vi "运维调试_总磷总氮.vi"() -> ()   [LabVIEW 2016, in "斯坦道总磷总氮.lvlib"]
uses:
  <vilib>/Utility/miscctls.llb/LVPointTypeDef.ctl
  <vilib>/Plasmionique/MB Master/MB_Master/MB_Master.lvclass
  <vilib>/ptbypt/NI_PtbyPt.lvlib
panel:
  out "步骤":u16
  out "seconds since 1Jan1904 2":timestamp
  out "seconds since 1Jan1904":timestamp
  in  "周期设置":bool
  in  "流程操作":bool
  out "消解压力":sgl format="%#.2f kPa"
  out "权限等级":string
  out "总步数":i32
  out "滑动杆":dbl(slide) caption="测试进度" scale=0.0..100.0
  out "试剂余量显示":sgl[][](graph)
  in  "仪器校准":bool
  in  "参数查询":bool
  out "简易步骤名称":string
  in  "温度曲线":bool
  in  "试剂余量":bool
  in  "灯值调整":bool
  out "固件版本号":string
  out "模块版本号":string
  out "注射器温度":sgl format="%#.2f ℃"
  out "消解温度":sgl format="%#.2f ℃"
  out "ADC":sgl
  out "F3":sgl format="%#.6f"
  out "F2":sgl format="%#.6f"
  out "F1":sgl format="%#.6f"
  out "F0":sgl format="%#.6f"
  out "运行状态":T1 {"数据时间:" format="%<%y/%m/%d %H:%M:%S>T"; "仪器时间:" format="%<%y/%m/%d %H:%M:%S>T"}
  in  "单选按钮":T2=enum."总氮"
  in  "布尔":bool
  in  "外设固件":bool
  out "字符串 2":string
  in  "数组":string[](array[string])
  in  "返回":bool
  in  "参数设置":bool
  out "集成报警信息":string
  in  "停止":bool
  in  "手动启动":bool
  in  "调试":bool
  out "多列列表框":i32(listbox)
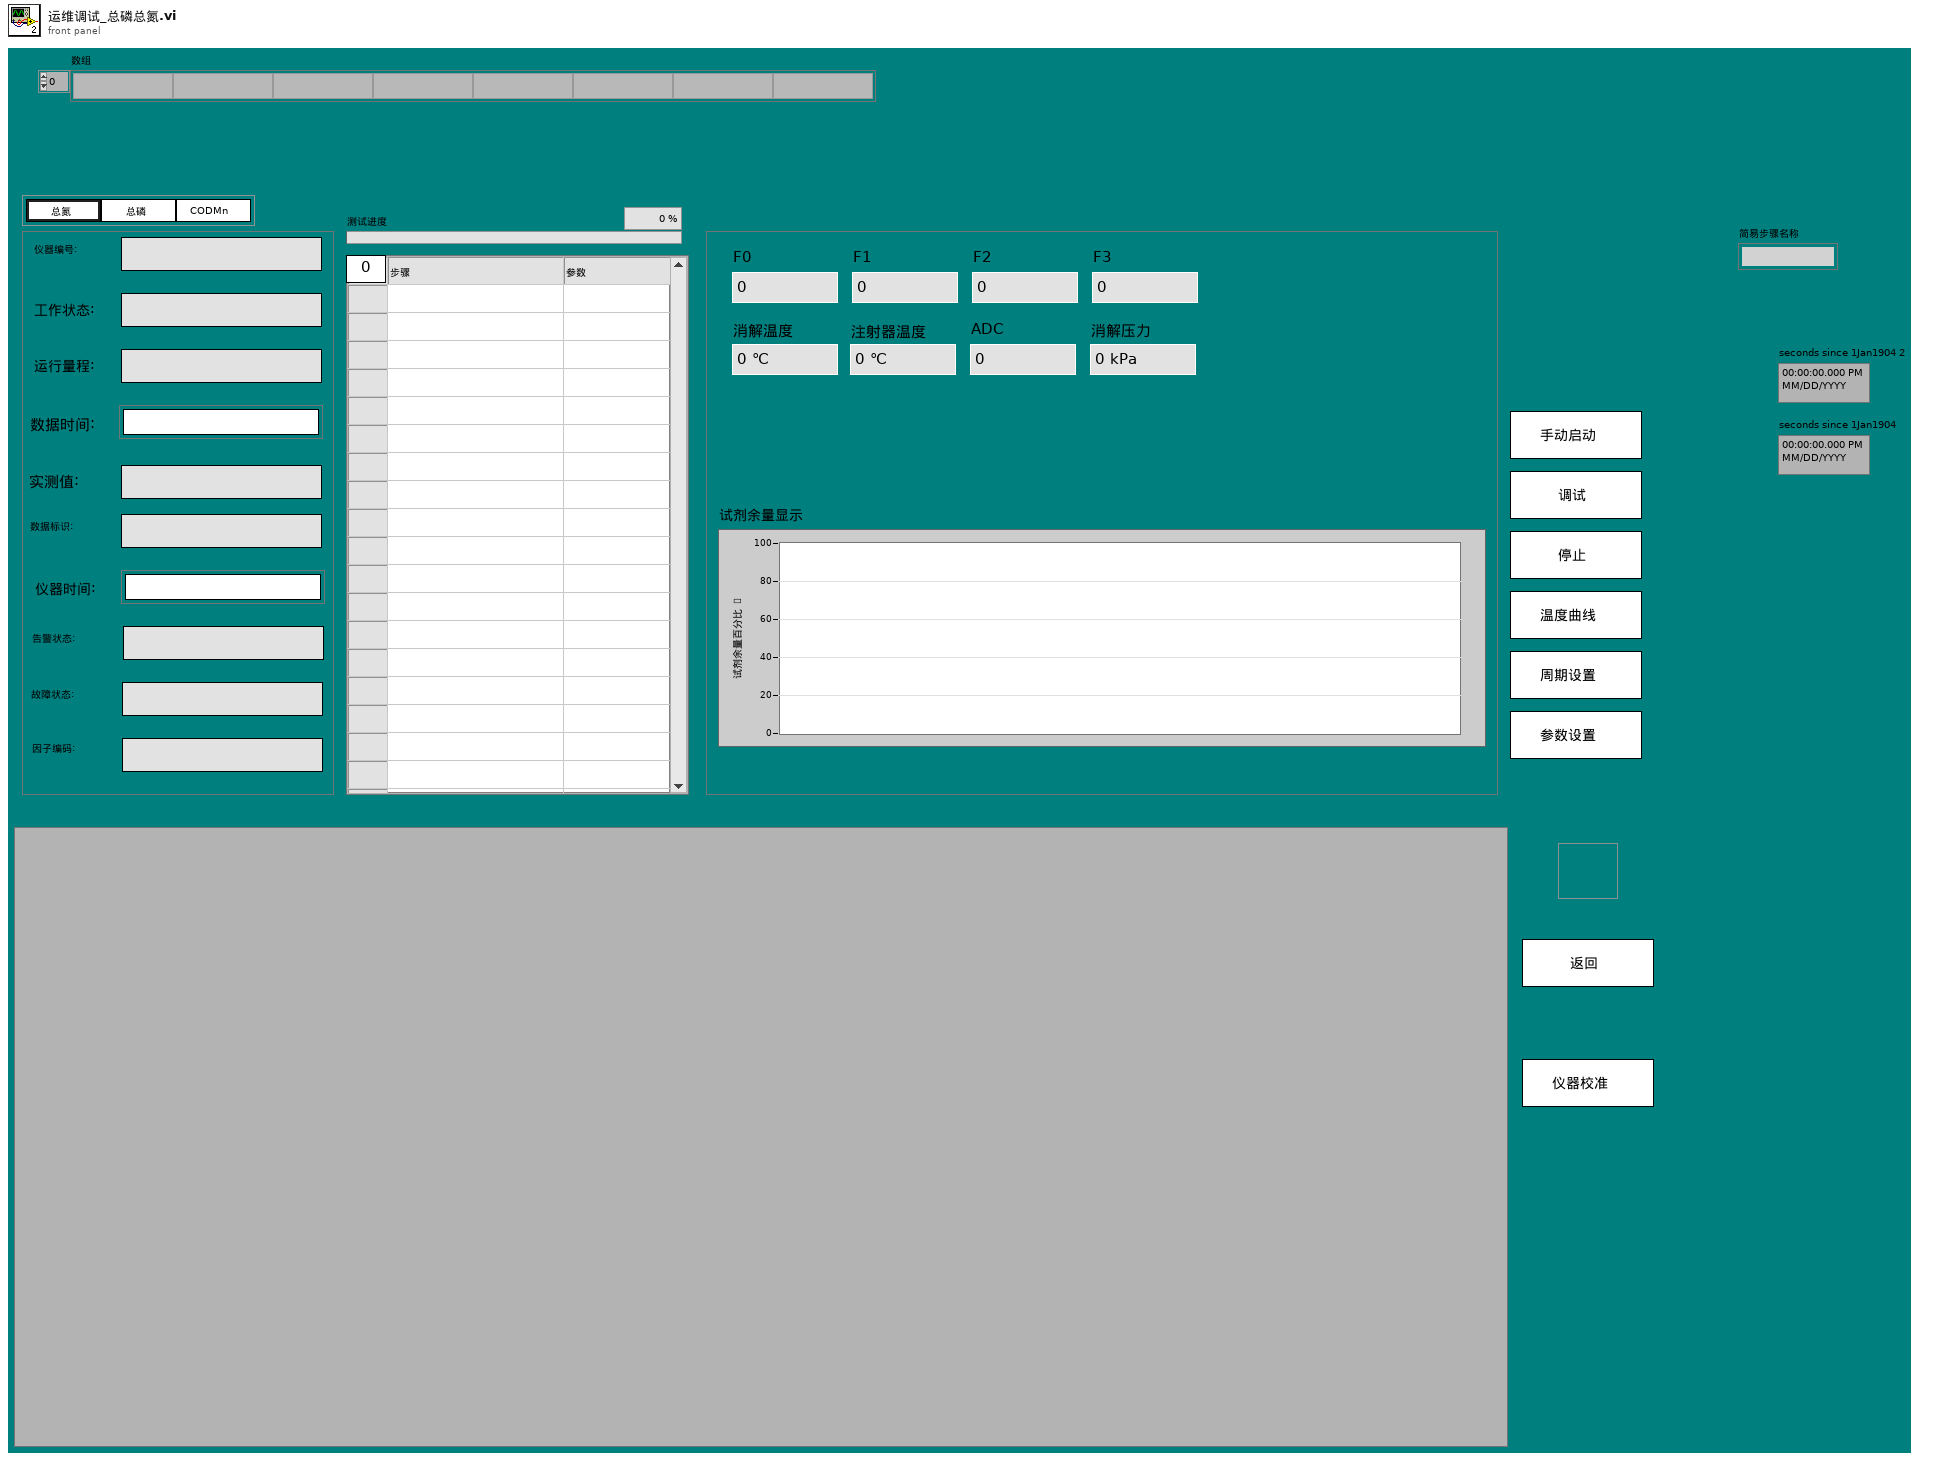
[diagram p1: front panel]
types:
  T1 = cluster{"仪器编号:":string, "工作状态:":string, "运行量程: ":string, "数据时间:":timestamp, "实测值:":string, "数据标识: ":string, "仪器时间:":timestamp, "告警状态: ":string, "故障状态:  ":string, "因子编码:":string}
  T2 = typedef "斯坦道总磷总氮.lvlib/启动参数显示控件.ctl" = enum32{"COD", "氨氮", "总氮", "总磷", "磷酸盐", "硝氮", "亚硝氮", "硅酸盐", "硫化物", "氟化物", "CODMn"}
  T3 = typedef "LVPointTypeDef.ctl" = cluster{"Horizontal":i16, "Vertical":i16}
  T4 = cluster{"系统时间":timestamp, "工作状态":u16, "测量模式":enum16{"待机", "连续模式", "周期模式", "定点模式", "受控模式", "手动模式"}, "告警代码":u16, "故障代码":u16, "日志代码":u16, "软件版本":u16, "F0":sgl, "F1":sgl, "F2":sgl, "F3":sgl, "T":sgl, "H":sgl, "id":u16, "flowid":u16, "量程":u16, "总磷控温温度1":sgl, "营养盐控温温度2":sgl, "ADC":sgl, "结果值":sgl, "运行时间":u16, "步骤详情":string, "步骤流程":string}
  T5 = typedef "报警信息字段定义.ctl" = cluster{"时间":timestamp, "参数":string, "元器件":string, "故障现象":string, "故障分析":string, "state":string, "code":string, "platform_alarm_code":string, "是否上报":string}
  T6 = typedef "Alarm interface.lvlib/报警短信语音交互.ctl" = cluster{"参数":string, "元器件":string, "故障现象":string, "code":string, "platform_alarm_code":string, "solutionList":cluster{"reason":string, "solution":string}[], "是否上报":string}
  T7 = cluster{"Major":u16, "Minor":u16, "Fix":u16, "Build":u16}
  T8 = typedef "LVStringsAndValuesArrayTypeDef_U16.ctl" = cluster{"String":string, "Value":u16}[]
  T9 = cluster{"因子编码":u32, "单位":u16, "标样参考值":sgl, "水样数据时间":timestamp, "水样实测值":sgl, "水样数据标识":string, "标样数据时间":timestamp, "标样实测值":sgl, "标样数据标识":string, "空白数据时间":timestamp, "空白实测值":sgl, "空白数据标识":string, "零点核查数据时间":timestamp, "零点核查实测值":sgl, "零点核查数据标识":string, "跨度核查数据时间":timestamp, "跨度核查实测值":sgl, "跨度核查数据标识":string, "加标回收数据时间":timestamp, "加标回收实测值":sgl, "加标回收数据标识":string, "平行样数据时间":timestamp, "平行样实测值":sgl, "平行样数据标识":string, "F0":sgl, "F1":sgl, "F2":sgl, "F3":sgl, "F4":sgl, "F5":sgl, "F6":sgl, "F7":sgl, "温度":sgl, "湿度":sgl, "X值":sgl, "fidrange":u16, "X1值":sgl}[]
  T10 = typedef "SingleStepTestV3.lvlib/SingleStepTestV3.lvclass/仪器版本.ctl" = enum16{"V3.1版", "V4版", "V3版", "V4.2版"}
  T11 = cluster{"因子编码":u32, "单位":u16, "标样参考值":sgl, "水样数据时间":timestamp, "水样实测值":sgl, "水样数据标识":string, "标样数据时间":timestamp, "标样实测值":sgl, "标样数据标识":string, "空白数据时间":timestamp, "空白实测值":sgl, "空白数据标识":string, "零点核查数据时间":timestamp, "零点核查实测值":sgl, "零点核查数据标识":string, "跨度核查数据时间":timestamp, "跨度核查实测值":sgl, "跨度核查数据标识":string, "加标回收数据时间":timestamp, "加标回收实测值":sgl, "加标回收数据标识":string, "平行样数据时间":timestamp, "平行样实测值":sgl, "平行样数据标识":string, "F0":sgl, "F1":sgl, "F2":sgl, "F3":sgl, "F4":sgl, "F5":sgl, "F6":sgl, "F7":sgl, "温度":sgl, "湿度":sgl, "X值":sgl, "fidrange":u16, "X1值":sgl}
  T12 = typedef "TimingControl.lvlib/TimingControl.lvclass/国标控制命令.ctl" = enum16{"启动测量", "标样核查", "零点核查", "跨度核查", "空白测试", "平行样测试", "加标回收", "空白校准", "标样校准", "初始化（清洗）", "停止测试", "仪器重启", "校时", "模式设置", "测量间隔设置"}
  T13 = typedef "TimingControl.lvlib/TimingControl.lvclass/测量参数.ctl" = u16
  T14 = enum32{"Bad", "Idle", "Run top level", "Running"}
  T15 = cluster{"时间标识":timestamp, "设备":string, "日志信息":string, "流程参数":string}
  T16 = typedef "LVRowAndColumnUnsignedTypeDef.ctl" = cluster{"Row":u32, "Column":u32}
  T17 = typedef "操作日志字段定义.ctl" = cluster{"时间":timestamp, "参数":string, "日志信息":string, "流程参数":string}
  T18 = cluster{"站号":u16, "量程切换":enum32{"H", "L", "AUTO"}, "控制命令":enum16{"启动测量", "标样核查", "零点核查", "跨度核查", "空白测试", "平行样测试", "加标回收", "空白校准", "标样校准", "初始化（清洗）", "停止测试", "仪器重启", "校时", "模式设置", "测量间隔设置"}, "模式设置":enum16{"待机", "连续模式", "周期模式", "定点模式", "受控模式", "手动模式"}, "测量间隔":u16}
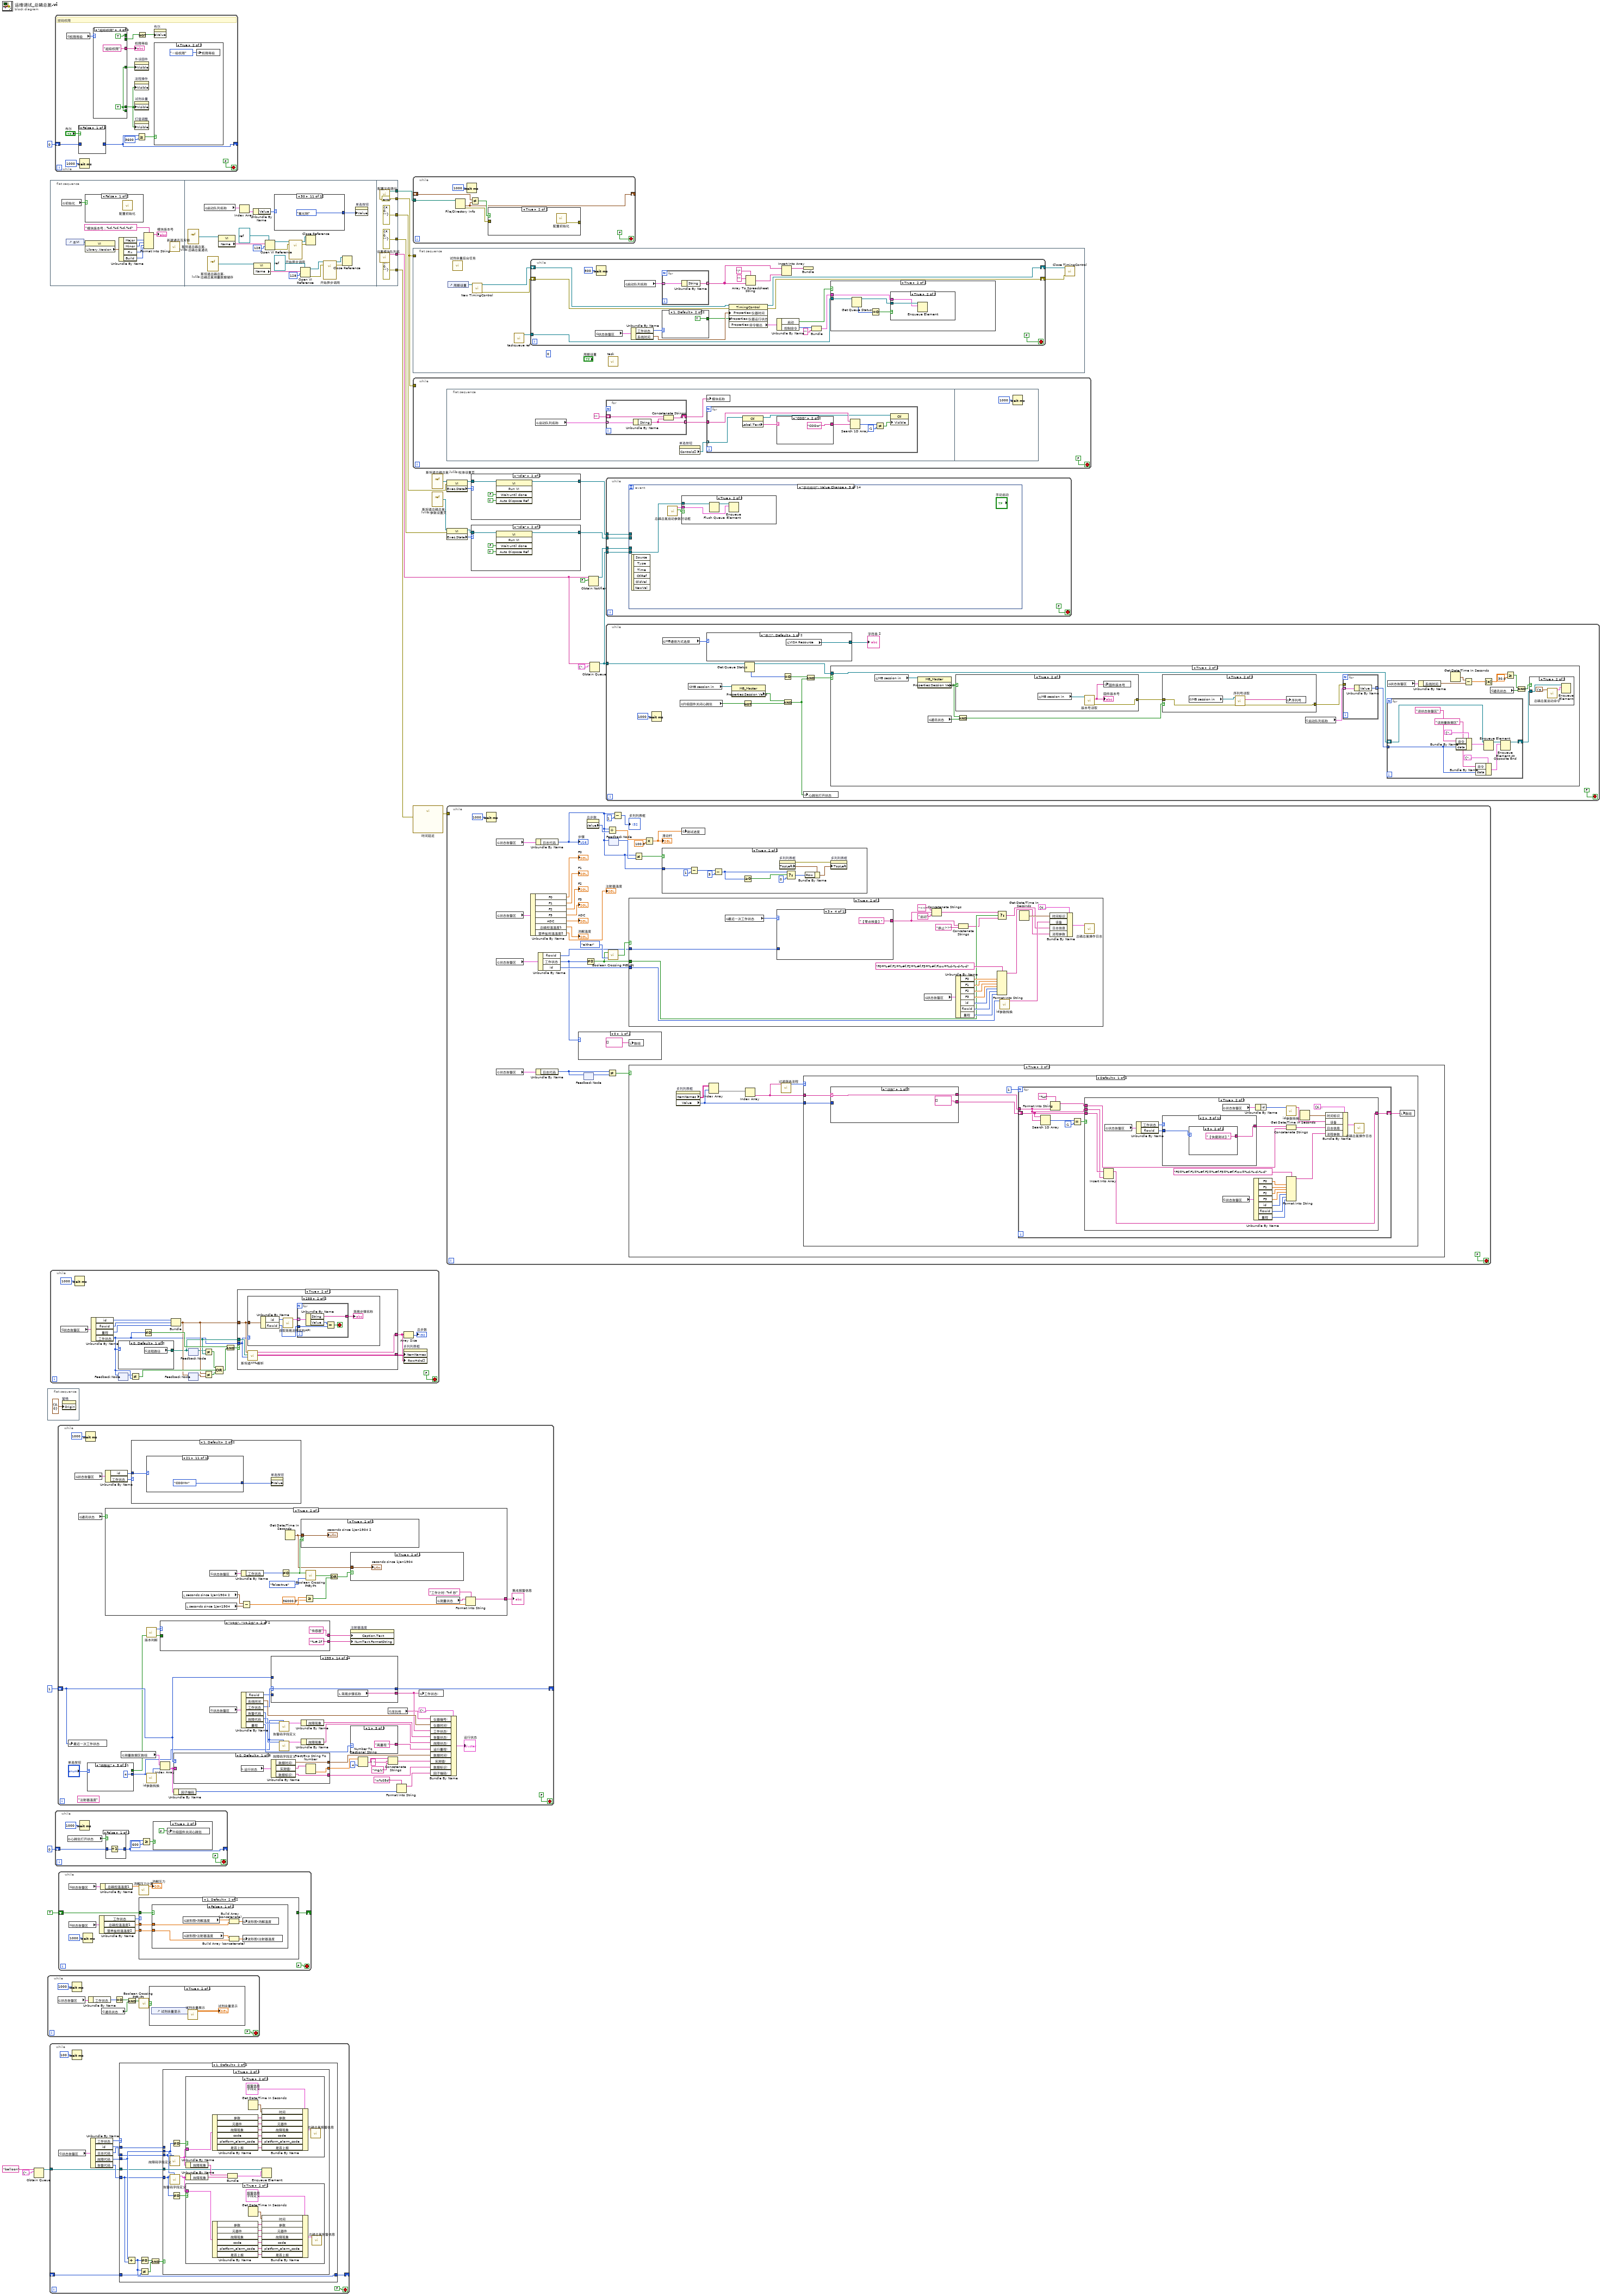
[diagram p0: block diagram]
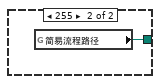
[diagram p6: hidden frame]
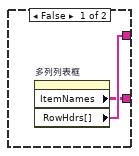
[diagram p7: hidden frame]
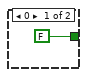
[diagram p11: hidden frame]
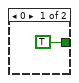
[diagram p18: hidden frame]
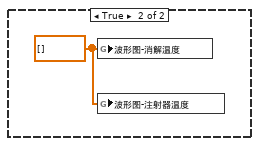
[diagram p19: hidden frame]
diagram:
  n1 = Obtain Queue(name (unnamed)="balloon" ("名称（未命名）"), element data type=cluster{"Title":string, "Body":string} {"Title"="", "Body"=""}) -> (queue out=w1:refnum<queue>)  [unwired: 3 in, 2 out]
  n2 = flat-sequence {
    frame #0 {
      n3 = property on="窗格" class="Pane"("Origin"=T3 {"Horizontal"=0, "Vertical"=0} ("原点")) -> ()  [unwired: 2 in, 2 out]
    }
  }
  n4 = while {
    stop <- FALSE stop-if-true
    n5 = global read "VAR总磷总氮全局变量.vi" "状态告警区"() -> (w32:T4)
    n6 = Wait (ms)(milliseconds to wait=u32 1000 ("等待时间（毫秒）")) -> ()  [unwired: 1 out]
    n7 = Unbundle By Name(w32) -> ("工作状态"=w30:u16)
    n8 = global read "VAR总磷总氮全局变量.vi" "通讯状态"() -> (w33:bool)
    n9 = Equal To 0?(x=w30) -> (x = 0?=w29:bool)
    n10 = And(x=w29, y=w33) -> (x .and. y?=w31:bool)
    n11 = call <vilib>:"Boolean Crossing PtByPt.vi"("input"=w31) -> ("crossing"=w28:bool)  [unwired: 2 in]
    n12 = case shown="True" w28 {
      frame False {
      }
      frame True {
        n13 = control-ref of="试剂余量显示"() -> (w36:refnum<vi>)
        n14 = call "试剂余量展示.vi"("波形图 2"=w36) -> ("波形图"=→"试剂余量显示":sgl[][])  [unwired: 10 in]
      }
    }
  }
  n15 = while {
    shift-right: [w40] -> _
    shift-left: _ -> [w42]
    tunnel: w1 -> [w39]
    stop <- FALSE stop-if-true
    n16 = global read "VAR总磷总氮全局变量.vi" "状态告警区"() -> (w38:T4)
    n17 = Wait (ms)(milliseconds to wait=u32 100 ("等待时间（毫秒）")) -> ()  [unwired: 1 out]
    n18 = Unbundle By Name(w38) -> ("工作状态"=w47:u16, "id"=w46:u16, "日志代码"=w45:u16, "故障代码"=w44:u16, "告警代码"=w43:u16)
    n19 = case shown="1, Default" w47 {
      tunnel: w46 -> [_ w51]
      tunnel: w45 -> [_ w54]
      tunnel: w44 -> [_ w53]
      tunnel: w43 -> [_ w52]
      tunnel: w42 -> [w49 w57]
      tunnel: [w49 w55] -> w40
      tunnel: w39 -> [_ w50]
      frame 0 {
      }
      frame 1, Default {
        n20 = Add(x=w53, y=w52) -> (x+y=w55:u16)
        n21 = Not Equal To 0?(x=w55) -> (x != 0?=w59:bool)
        n22 = Not Equal?(x=w55, y=w57) -> (x != y?=w58:bool)
        n23 = And(x=w59, y=w58) -> (x .and. y?=w56:bool)
        n24 = case shown="True" w56 {
          tunnel: w54 -> [_ _]
          tunnel: w53 -> [_ w62]
          tunnel: w52 -> [_ w61]
          tunnel: w51 -> [_ w63]
          tunnel: w50 -> [_ w68]
          frame False {
          }
          frame True {
            n25 = call "故障码字段定义.vi"("id"=w63, "故障代码"=w62) -> ("告警信息"=w64:T6)  [unwired: 9 in]
            n26 = call "告警码字段定义.vi"("id"=w63, "告警代码"=w61) -> ("告警信息"=w60:T6)  [unwired: 9 in]
            n27 = Not Equal To 0?(x=w62) -> (x != 0?=w66:bool)
            n28 = Not Equal To 0?(x=w61) -> (x != 0?=w65:bool)
            n29 = case shown="True" w66 {
              tunnel: w64 -> [_ w88]
              frame False {
              }
              frame True {
                n30 = Unbundle By Name(w88) -> ("参数"=w87:string, "元器件"=w86:string, "故障现象"=w85:string, "code"=w84:string, "platform_alarm_code"=w83:string, "是否上报"=w82:string)
                n31 = Get Date/Time In Seconds() -> (seconds since 1Jan1904=w89:timestamp)
                n32 = Bundle By Name(cluster=T5 {"时间"=timestamp(0 s since 1904-01-01), "参数"="", "元器件"="", "故障现象"="", "故障分析"="", "state"="", "code"="", "platform_alarm_code"="", "是否上报"=""} ("data in"), "时间"=w89, "参数"=w87, "元器件"=w86, "故障现象"=w85, "code"=w84, "platform_alarm_code"=w83, "是否上报"=w82) -> (w81:T5)
                n33 = call "总磷总氮报警信息.vi"("data in"=w81) -> ()  [unwired: 10 in, 1 out]
              }
            }
            n34 = Unbundle By Name(w64) -> ("故障现象"=w70:string)
            n35 = Unbundle By Name(w60) -> ("故障现象"=w69:string)
            n36 = case shown="True" w65 {
              tunnel: w60 -> [_ w72]
              frame False {
              }
              frame True {
                n37 = Unbundle By Name(w72) -> ("参数"=w75:string, "元器件"=w76:string, "故障现象"=w77:string, "code"=w78:string, "platform_alarm_code"=w79:string, "是否上报"=w80:string)
                n38 = Get Date/Time In Seconds() -> (seconds since 1Jan1904=w74:timestamp)
                n39 = Bundle By Name(cluster=T5 {"时间"=timestamp(0 s since 1904-01-01), "参数"="", "元器件"="", "故障现象"="", "故障分析"="", "state"="", "code"="", "platform_alarm_code"="", "是否上报"=""} ("data in"), "时间"=w74, "参数"=w75, "元器件"=w76, "故障现象"=w77, "code"=w78, "platform_alarm_code"=w79, "是否上报"=w80) -> (w71:T5)
                n40 = call "总磷总氮报警信息.vi"("data in"=w71) -> ()  [unwired: 10 in, 1 out]
              }
            }
            n41 = Bundle("故障现象"=w70, "故障现象"=w69) -> (w67:cluster{"故障现象":string, "故障现象":string})  [unwired: 1 in]
            n42 = Enqueue Element(queue=w68, element=w67) -> ()  [unwired: 2 in, 3 out]
          }
        }
      }
    }
  }
  n43 = flat-sequence {
    tunnel: [w137] -> w20
    tunnel: [errorcluster {"status"=FALSE, "code"=0, "source"=""} ("错误输入（无错误）")] -> w11
    tunnel: [errorcluster {"status"=FALSE, "code"=0, "source"=""} ("错误输入（无错误）")] -> w10
    tunnel: [w134] -> w8
    tunnel: [errorcluster {"status"=FALSE, "code"=0, "source"=""} ("error out")] -> w7
    tunnel: [errorcluster {"status"=FALSE, "code"=0, "source"=""} ("错误输入（无错误）")] -> w6
    frame #0 {
      n44 = global read "VAR总磷总氮全局变量.vi" "初始化"() -> (w91:bool)
      n45 = control-ref of="本VI"() -> (w99:refnum<vi>)
      n46 = case shown="False" w91 {
        frame False {
          n47 = call "配置初始化.vi"() -> ()  [unwired: 11 in, 1 out]
        }
        frame True {
        }
      }
      n48 = property class="VI"(reference=w99) -> ("Library.Version"=w98:T7)  [unwired: 1 in, 2 out]
      n49 = Unbundle By Name(w98) -> ("Major"=w96:u16, "Minor"=w95:u16, "Fix"=w94:u16, "Build"=w93:u16)
      n50 = Format Into String(format string="模块版本号：%d.%d.%d.%d" ("格式字符串"), w96, w95, w94, w93) -> (resulting string=→"模块版本号":string)  [unwired: 2 in, 1 out]
      n51 = call "新建通讯互斥锁.vi"() -> ()  [unwired: 11 in, 1 out]
    }
    frame #1 {
      n52 = vi-ref "斯坦道总磷总氮.lvlib:总磷总氮通讯.vi"() -> (w104:refnum<vi>)
      n53 = global read "model config var.vi" "启动队列名称"() -> (w102:cluster{"String":string, "Value":u16}[])
      n54 = vi-ref "斯坦道总磷总氮.lvlib:总磷总氮测量数据储存.vi"() -> (w112:refnum<vi>)
      n55 = property class="VI"(reference=w104) -> ("Name"=w105:string)  [unwired: 1 in, 2 out]
      n56 = Index Array(array=w102) -> (element=w101:cluster{"String":string, "Value":u16})  [unwired: 1 in]
      n57 = Unbundle By Name(w101) -> ("Value"=w100:u16)
      n58 = property class="VI"(reference=w112) -> ("Name"=w119:string)  [unwired: 1 in, 2 out]
      n59 = Open VI Reference(type specifier VI Refnum (for type only)=refnum<vi> refnum, vi path=w105, options=128 ("选项")) -> (vi reference=w107:refnum<vi>, error out=w109:errorcluster)  [unwired: 3 in]
      n60 = case shown="50" w100 {
        tunnel: [w120 启动参数显示控件."总磷" ("单选按钮") 启动参数显示控件."总氮" ("单选按钮") 启动参数显示控件."COD" ("单选按钮") 启动参数显示控件."氨氮" ("单选按钮") 启动参数显示控件."磷酸盐" ("单选按钮") 启动参数显示控件."硝氮" ("单选按钮") 启动参数显示控件."亚硝氮" ("单选按钮") 启动参数显示控件."硅酸盐" ("单选按钮") 启动参数显示控件."硫化物" ("单选按钮") 启动参数显示控件."氟化物" ("单选按钮") 启动参数显示控件."CODMn" ("单选按钮")] -> w103
        frame 0, Default {
          n61 = property on="单选按钮" class="RadioBtnsControl (strict)"() -> ("Value"=w120:T2)  [unwired: 2 in, 2 out]
        }
        frame 1 {
        }
        frame 2 {
        }
        frame 22 {
        }
        frame 3 {
        }
        frame 4 {
        }
        frame 5 {
        }
        frame 6 {
        }
        frame 7 {
        }
        frame 8 {
        }
        frame 50 {
        }
        frame 21 {
        }
      }
      n62 = call-by-ref "开始异步调用"(reference=w107, error in=w109) -> (reference out=w111:refnum<vi>, error out=w110:errorcluster)  [unwired: 12 in]
      n63 = Open VI Reference(type specifier VI Refnum (for type only)=refnum<vi> refnum, vi path=w119, options=128 ("选项")) -> (vi reference=w117:refnum<vi>, error out=w115:errorcluster)  [unwired: 3 in]
      n64 = Close Reference(reference=w111, error in (no error)=w110) -> ()  [unwired: 1 out]
      n65 = call-by-ref "开始异步调用"(reference=w117, error in=w115) -> (reference out=w113:refnum<vi>, error out=w114:errorcluster)  [unwired: 12 in]
      n66 = Close Reference(reference=w113, error in (no error)=w114) -> ()  [unwired: 1 out]
      n67 = property on="单选按钮" class="RadioBtnsControl (strict)"("Value"=w103) -> ()  [unwired: 2 in, 2 out]
    }
    frame #2 {
      n68 = call "配置文件路径.vi"() -> ("appended path"=w134:path)  [unwired: 11 in]
      n69 = call "设置模块队列名.vi"() -> ("Msg"=w137:string)  [unwired: 5 in]
    }
  }
  n70 = while {
    stop <- FALSE stop-if-true
    n71 = global read "VAR总磷总氮全局变量.vi" "状态告警区"() -> (w149:T4)
    n72 = Wait (ms)(milliseconds to wait=u32 1000 ("等待时间（毫秒）")) -> ()  [unwired: 1 out]
    n73 = Unbundle By Name(w149) -> ("id"=w148:u16, "flowid"=w147:u16, "量程"=w146:u16, "工作状态"=w139:u16)
    n74 = case shown="0, Default" w139 {
      tunnel: [w159 w160] -> w141
      frame 0, Default {
        n75 = global read "总磷总氮断电保存全局变量.vi" "流程路径"() -> (w159:path)
      }
      frame 255 {
        n76 = global read "总磷总氮断电保存全局变量.vi" "简易流程路径"() -> (w160:path)
      }
    }
    n77 = feedback #1() -> (w138:u16)  [unwired: 1 in]
    n78 = feedback-in #1(w139) -> ()
    n79 = Not Equal?(x=w138, y=w139) -> (x != y?=w155:bool)
    n80 = Not Equal To 0?(x=w139) -> (x != 0?=w150:bool)
    n81 = Bundle("id"=w148, "flowid"=w147, "量程"=w146) -> (w143:cluster{"id":u16, "flowid":u16, "量程":u16})  [unwired: 1 in]
    n82 = feedback #2() -> (w140:path)  [unwired: 1 in]
    n83 = feedback-in #2(w141) -> ()
    n84 = feedback-in #3(w143) -> ()
    n85 = feedback #3() -> (w144:cluster{"id":u16, "flowid":u16, "量程":u16})  [unwired: 1 in]
    n86 = Not Equal?(x=w140, y=w141) -> (x != y?=w154:bool)
    n87 = Not Equal?(x=w143, y=w144) -> (x != y?=w142:bool)
    n88 = Compound Arithmetic op=OR ("复合运算")(w154, w155, w142) -> (w156:bool)
    n89 = And(x=w150, y=w156) -> (x .and. y?=w151:bool)
    n90 = case shown="True" w151 {
      tunnel: [w162 w165] -> w153
      tunnel: [w161 w166] -> w157
      tunnel: w143 -> [_ w164]
      tunnel: w141 -> [_ w167]
      tunnel: w139 -> [_ w163]
      frame False {
        n91 = property on="多列列表框" class="MCListbox (strict)"() -> ("ItemNames"=w161:string[][], "RowHdrs[]"=w162:string[])  [unwired: 2 in, 2 out]
      }
      frame True {
        n92 = case shown="255" w163 {
          tunnel: w164 -> [_ w172]
          frame 0, Default {
          }
          frame 255 {
            n93 = Unbundle By Name(w172) -> ("id"=w171:u16, "flowid"=w169:u16)
            n94 = call "获取简易流程名称API.vi"("参数下拉列表"=w171) -> ("字符串与值[]"=w170:T8)  [unwired: 9 in, 1 out]
            n95 = for {
              tunnel: w170 -> [w177] mode=indexing
              tunnel: w169 -> [w175]
              tunnel: [w174] -> w168
              stop <- w173 stop-if-true
              n96 = Unbundle By Name(w177) -> ("String"=w174:string, "Value"=w176:u16)
              n97 = Equal?(x=w176, y=w175) -> (x = y?=w173:bool)
            }
            "简易步骤名称" <- w168
          }
        }
        n98 = call "斯坦道XML解析.vi"("工作状态"=w163, "添加的路径"=w167, "参数簇"=w164) -> ("步骤名"=w166:string[][], "索引"=w165:string[])  [unwired: 6 in, 1 out]
      }
    }
    n99 = Array Size(array=w153) -> (size(s)=→"总步数":i32)
    n100 = property on="多列列表框" class="MCListbox (strict)"("ItemNames"=w157, "RowHdrs[]"=w153) -> ()  [unwired: 2 in, 2 out]
  }
  n101 = while {
    shift-right: [w187] -> _
    shift-left: u32 0 ("y") -> [w189]
    stop <- FALSE stop-if-true
    # "密码权限"
    n102 = global read "VAR总磷总氮全局变量.vi" "权限等级"() -> (w184:enum16{"一级权限", "二级权限", "三级权限", "超级权限"})
    n103 = case shown="False" "布尔" {
      tunnel: w189 -> [_ w202]
      tunnel: [_ w201] -> w187
      frame False {
      }
      frame True {
        n104 = Increment(x=w202) -> (x+1=w201:u32)
      }
    }
    n105 = Wait (ms)(milliseconds to wait=u32 1000 ("等待时间（毫秒）")) -> ()  [unwired: 1 out]
    n106 = case shown="\"超级权限\"" w184 {
      tunnel: [_ w194 w196 w199] -> w178
      tunnel: [_ _ w196 w199] -> _
      tunnel: [_ w194 w196 w199] -> w183
      tunnel: [_ _ _ TRUE] -> _
      tunnel: [TRUE _ _ _] -> w181
      tunnel: ["一级权限" "二级权限" "三级权限" "超级权限"] -> w179
      frame "一级权限", Default {
      }
      frame "二级权限" {
        w194 = TRUE
      }
      frame "三级权限" {
        w196 = TRUE
      }
      frame "超级权限" {
        w199 = TRUE
      }
    }
    "权限等级" <- w179
    n107 = property on="外设固件" class="Bool"("Visible"=w183) -> ()  [unwired: 2 in, 2 out]
    n108 = property on="流程操作" class="Bool"("Visible"=w178) -> ()  [unwired: 2 in, 2 out]
    n109 = property on="试剂余量" class="Bool"("Visible"=w178) -> ()  [unwired: 2 in, 2 out]
    n110 = property on="灯值调整" class="Bool"("Visible"=w178) -> ()  [unwired: 2 in, 2 out]
    n111 = Greater Or Equal?(x=w187, y=u32 3600) -> (x >= y?=w185:bool)
    n112 = Not(x=w181) -> (.not. x?=w180:bool)
    n113 = property on="布尔" class="Bool (strict)"("Value"=w180) -> ()  [unwired: 2 in, 2 out]
    n114 = case shown="True" w185 {
      frame False {
      }
      frame True {
        n115 = global write "VAR总磷总氮全局变量.vi" "权限等级"(enum16{"一级权限", "二级权限", "三级权限", "超级权限"}."一级权限" ("权限等级")) -> ()
      }
    }
  }
  n116 = while {
    shift-right: [w207] -> _
    shift-left: 0 -> [w208]
    stop <- FALSE stop-if-true
    n117 = global read "VAR总磷总氮全局变量.vi" "心跳包打开状态"() -> (w203:bool)
    n118 = Wait (ms)(milliseconds to wait=u32 1000 ("等待时间（毫秒）")) -> ()  [unwired: 1 out]
    n119 = case shown="False" w203 {
      tunnel: w208 -> [w212 _]
      tunnel: [w211 _] -> w207
      frame False {
        n120 = Increment(x=w212) -> (x+1=w211:i32)
      }
      frame True {
      }
    }
    n121 = Greater Or Equal?(x=w207, y=600) -> (x >= y?=w205:bool)
    n122 = case shown="True" w205 {
      frame False {
      }
      frame True {
        n123 = global write "VAR总磷总氮全局变量.vi" "升级固件关闭心跳包"(FALSE ("关闭心跳包")) -> ()
      }
    }
  }
  n124 = while {
    shift-right: [w224] -> _
    shift-left: u16 1 ("工作状态") -> [w222]
    stop <- FALSE stop-if-true
    (unwired) "注射器温度"
    n125 = global write "VAR总磷总氮全局变量.vi" "最近一次工作状态"(w222) -> ()
    n126 = global read "VAR总磷总氮全局变量.vi" "状态告警区"() -> (w244:T4)
    n127 = global read "VAR总磷总氮全局变量.vi" "通讯状态"() -> (w255:bool)
    n128 = Wait (ms)(milliseconds to wait=u32 1000 ("等待时间（毫秒）")) -> ()  [unwired: 1 out]
    n129 = case shown="\"磷酸盐\"" "单选按钮" {
      tunnel: [22 3 2 1 4 5 6 7 8 50 21] -> w213
      tunnel: [_ TRUE _ _ _ _ _ _ _ _ _] -> w216
      frame "COD", Default {
      }
      frame "氨氮" {
      }
      frame "总氮" {
      }
      frame "总磷" {
      }
      frame "磷酸盐" {
      }
      frame "硝氮" {
      }
      frame "亚硝氮" {
      }
      frame "硅酸盐" {
      }
      frame "硫化物" {
      }
      frame "氟化物" {
      }
      frame "CODMn" {
      }
    }
    n130 = Unbundle By Name(w244) -> ("id"=w243:u16, "工作状态"=w239:u16)
    n131 = case shown="True" w255 {
      tunnel: ["通讯异常" ("集成报警信息") w374] -> w254
      frame False {
      }
      frame True {
        n132 = local read "seconds since 1Jan1904 2"() -> (w366:timestamp)
        n133 = local read "seconds since 1Jan1904"() -> (w369:timestamp)
        n134 = global read "VAR总磷总氮全局变量.vi" "状态告警区"() -> (w376:T4)
        n135 = Unbundle By Name(w376) -> ("工作状态"=w372:u16)
        n136 = Subtract(x=w366, y=w369) -> (x-y=w365:dbl)
        n137 = Not Equal To 0?(x=w372) -> (x != 0?=w368:bool)
        n138 = Get Date/Time In Seconds() -> (seconds since 1Jan1904=w367:timestamp)
        n139 = case shown="True" w368 {
          tunnel: w367 -> [_ w377]
          frame False {
          }
          frame True {
            "seconds since 1Jan1904 2" <- w377
          }
        }
        n140 = Greater Or Equal?(x=w365, y=36000.0) -> (x >= y?=w362:bool)
        n141 = call <vilib>:"Boolean Crossing PtByPt.vi"("direction"=enum16{"either", "false-true", "true-false"}."false-true", "input"=w368) -> ("crossing"=w370:bool)  [unwired: 1 in]
        n142 = Or(x=w370, y=w362) -> (x .or. y?=w363:bool)
        n143 = case shown="True" w363 {
          tunnel: w367 -> [_ w378]
          frame False {
          }
          frame True {
            "seconds since 1Jan1904" <- w378
          }
        }
        n144 = global read "VAR总磷总氮全局变量.vi" "测量状态"() -> (w373:string)
        n145 = Format Into String(format string="工作计时: %d 秒" ("格式字符串"), initial string=w373, w365) -> (resulting string=w374:string)  [unwired: 1 in, 1 out]
      }
    }
    "集成报警信息" <- w254
    n146 = global read "VAR总磷总氮全局变量.vi" "测量数据区数组"() -> (w228:T9)
    n147 = case shown="1, Default" w239 {
      tunnel: w243 -> [_ w311]
      frame 0 {
      }
      frame 1, Default {
        n148 = case shown="21" w311 {
          tunnel: [w312 启动参数显示控件."总磷" ("单选按钮") 启动参数显示控件."总氮" ("单选按钮") 启动参数显示控件."COD" ("单选按钮") 启动参数显示控件."氨氮" ("单选按钮") 启动参数显示控件."磷酸盐" ("单选按钮") 启动参数显示控件."硝氮" ("单选按钮") 启动参数显示控件."亚硝氮" ("单选按钮") 启动参数显示控件."硅酸盐" ("单选按钮") 启动参数显示控件."硫化物" ("单选按钮") 启动参数显示控件."CODMn" ("单选按钮") 启动参数显示控件."氟化物" ("单选按钮")] -> w310
          frame 0, Default {
            n149 = property on="单选按钮" class="RadioBtnsControl (strict)"() -> ("Value"=w312:T2)  [unwired: 2 in, 2 out]
          }
          frame 1 {
          }
          frame 2 {
          }
          frame 22 {
          }
          frame 3 {
          }
          frame 4 {
          }
          frame 5 {
          }
          frame 6 {
          }
          frame 7 {
          }
          frame 8 {
          }
          frame 21 {
          }
          frame 50 {
          }
        }
        n150 = property on="单选按钮" class="RadioBtnsControl (strict)"("Value"=w310) -> ()  [unwired: 2 in, 2 out]
      }
    }
    n151 = call "版本判断.vi"() -> ("仪器版本"=w218:T10)  [unwired: 11 in]
    n152 = call "id参数转换.vi"("id"=w213) -> ("数组资源索引"=w225:i32)  [unwired: 9 in, 1 out]
    n153 = case shown="\"V4版\", \"V4.2版\"" w218 {
      tunnel: [w258 "传感器" ("标题.文本")] -> w215
      tunnel: ["%#.2f ℃" ("数值文本.格式字符串") "%#.2f " ("数值文本.格式字符串")] -> w217
      tunnel: w216 -> [w261 _]
      frame "V3.1版", Default {
        n154 = Select(t="显色温度", s=w261, f="注射器温度" ("标题.文本")) -> (s? t:f=w258:string)
      }
      frame "V4版", "V4.2版" {
      }
    }
    n155 = Index Array(array=w228, index=w225) -> (element=w227:T11)
    n156 = case shown="0, Default" w222 {
      tunnel: [w279 w285 w289 w293 w297 w301 w305 w309] -> w238
      tunnel: [w277 w284 w288 w292 w295 w300 w304 w308] -> w233
      tunnel: [w280 w283 w287 w291 w294 w299 w303 w307] -> w231
      tunnel: w227 -> [_ w282 w286 w290 w296 w298 w302 w306]
      frame 0, Default {
        n157 = local read "运行状态"() -> (w281:T1)
        n158 = Unbundle By Name(w281) -> ("数据时间:"=w279:timestamp, "实测值:"=w278:string, "数据标识:"=w280:string)
        n159 = Fract/Exp String To Number(string=w278) -> (number=w277:dbl)  [unwired: 3 in, 1 out]
      }
      frame 1 {
        n160 = Unbundle By Name(w282) -> ("水样数据时间"=w285:timestamp, "水样实测值"=w284:sgl, "水样数据标识"=w283:string)
      }
      frame 2, 9 {
        n161 = Unbundle By Name(w286) -> ("标样数据时间"=w289:timestamp, "标样实测值"=w288:sgl, "标样数据标识"=w287:string)
      }
      frame 3 {
        n162 = Unbundle By Name(w290) -> ("零点核查数据时间"=w293:timestamp, "零点核查实测值"=w292:sgl, "零点核查数据标识"=w291:string)
      }
      frame 4 {
        n163 = Unbundle By Name(w296) -> ("跨度核查数据时间"=w297:timestamp, "跨度核查实测值"=w295:sgl, "跨度核查数据标识"=w294:string)
      }
      frame 7 {
        n164 = Unbundle By Name(w298) -> ("加标回收数据时间"=w301:timestamp, "加标回收实测值"=w300:sgl, "加标回收数据标识"=w299:string)
      }
      frame 5, 8 {
        n165 = Unbundle By Name(w302) -> ("空白数据时间"=w305:timestamp, "空白实测值"=w304:sgl, "空白数据标识"=w303:string)
      }
      frame 6 {
        n166 = Unbundle By Name(w306) -> ("平行样数据时间"=w309:timestamp, "平行样实测值"=w308:sgl, "平行样数据标识"=w307:string)
      }
    }
    n167 = Unbundle By Name(w227) -> ("因子编码"=w229:u32)
    n168 = global read "VAR总磷总氮全局变量.vi" "状态告警区"() -> (w253:T4)
    n169 = Unbundle By Name(w253) -> ("flowid"=w221:u16, "系统时间"=w249:timestamp, "工作状态"=w248:u16, "告警代码"=w242:u16, "故障代码"=w241:u16, "量程"=w247:u16)
    n170 = case shown="255" w248 {
      selector: w248 -> [w328 _ w334 w338 w341 w343 w345 w347 w349 w351 w353 w355 w357 w360]
      tunnel: [w329 "空闲" ("工作状态") "水样测量" ("工作状态") w337 "零点核查" ("工作状态") "跨度核查" ("工作状态") "空白测试" ("工作状态") "平行样测试" ("工作状态") "加标回收" ("工作状态") "空白校准" ("工作状态") "标样校准" ("工作状态") "初始化" ("工作状态") "单步调试" ("工作状态") w359] -> w223
      tunnel: [w327 w332 w334 w338 w341 w343 w345 w347 w349 w351 w353 w355 w357 w360] -> w224
      tunnel: w222 -> [w327 w332 _ _ _ _ _ _ _ _ _ _ _ _]
      tunnel: w221 -> [_ _ _ w336 _ _ _ _ _ _ _ _ _ _]
      frame Default {
        n171 = Format Into String(format string="%d" ("格式字符串"), initial string="未知" ("工作状态"), w328) -> (resulting string=w329:string)  [unwired: 1 in, 1 out]
      }
      frame 0 {
      }
      frame 1 {
      }
      frame 2 {
        n172 = case shown="5" w336 {
          tunnel: ["标样核查" ("工作状态") "快捷测试" ("工作状态")] -> w337
          frame 0, Default {
          }
          frame 5 {
          }
        }
      }
      frame 3 {
      }
      frame 4 {
      }
      frame 5 {
      }
      frame 6 {
      }
      frame 7 {
      }
      frame 8 {
      }
      frame 9 {
      }
      frame 10 {
      }
      frame 254 {
      }
      frame 255 {
        n173 = local read "简易步骤名称"() -> (w359:string)
      }
    }
    n174 = call "告警码字段定义.vi"("id"=w213, "告警代码"=w242) -> ("告警信息"=w220:T6)  [unwired: 9 in]
    n175 = call "故障码字段定义.vi"("id"=w213, "故障代码"=w241) -> ("告警信息"=w240:T6)  [unwired: 9 in]
    n176 = Unbundle By Name(w220) -> ("故障现象"=w219:string)
    n177 = Unbundle By Name(w240) -> ("故障现象"=w214:string)
    n178 = property on="注射器温度" class="DigNum (strict)"("Caption.Text"=w215, "NumText.FormatString"=w217) -> ()  [unwired: 2 in, 2 out]
    n179 = case shown="1" w247 {
      tunnel: ["" ("字符串") "低量程 " ("字符串") "高量程 " ("字符串")] -> w246
      frame Default {
      }
      frame 0 {
      }
      frame 1 {
      }
    }
    n180 = Number To Fractional String(number=w233, precision (6)=i16 4 ("精度(6)")) -> (F-format string=w235:string)  [unwired: 2 in]
    n181 = Concatenate Strings(w235, " " ("字符串"), "mg/L" ("字符串")) -> (w232:string)
    n182 = global read "VAR总磷总氮全局变量.vi" "序列号"() -> (w250:string)
    n183 = Format Into String(format string="w%05d" ("格式字符串"), w229) -> (resulting string=w245:string)  [unwired: 2 in, 1 out]
    n184 = global write "VAR总磷总氮全局变量.vi" "工作状态:"(w223) -> ()
    n185 = Bundle By Name(cluster=T1 {"仪器编号:"="", "工作状态:"="", "运行量程: "="", "数据时间:"=timestamp(0 s since 1904-01-01), "实测值:"="", "数据标识: "="", "仪器时间:"=timestamp(0 s since 1904-01-01), "告警状态: "="", "故障状态:  "="", "因子编码:"=""} ("运行状态"), "仪器编号:"=w250, "仪器时间:"=w249, "工作状态:"=w223, "告警状态:"=w219, "故障状态:"=w214, "运行量程:"=w246, "数据时间:"=w238, "实测值:"=w232, "数据标识:"=w231, "因子编码:"=w245) -> (→"运行状态":T1)
  }
  n186 = while {
    shift-right: [w380] -> _
    shift-left: TRUE -> [w381]
    stop <- FALSE stop-if-true
    n187 = global read "VAR总磷总氮全局变量.vi" "状态告警区"() -> (w384:T4)
    n188 = global read "VAR总磷总氮全局变量.vi" "状态告警区"() -> (w387:T4)
    n189 = Wait (ms)(milliseconds to wait=u32 1000 ("等待时间（毫秒）")) -> ()  [unwired: 1 out]
    n190 = Unbundle By Name(w387) -> ("工作状态"=w382:u16, "总磷控温温度1"=w386:sgl, "营养盐控温温度2"=w385:sgl)
    n191 = Unbundle By Name(w384) -> ("总磷控温温度1"=w383:sgl)
    n192 = call "消解压力计算.vi"("当前消解温度"=w383) -> ("消解压力"=→"消解压力":dbl)  [unwired: 10 in]
    n193 = case shown="1, Default" w382 {
      tunnel: w386 -> [_ w393]
      tunnel: w385 -> [_ w392]
      tunnel: w381 -> [_ w391]
      tunnel: [TRUE _] -> w380
      frame 0 {
      }
      frame 1, Default {
        n194 = case shown="False" w391 {
          tunnel: w393 -> [w399 _]
          tunnel: w392 -> [w398 _]
          frame False {
            n195 = global read "VAR总磷总氮全局变量.vi" "波形图-消解温度"() -> (w397:sgl[])
            n196 = global read "VAR总磷总氮全局变量.vi" "波形图-注射器温度"() -> (w396:sgl[])
            n197 = Build Array (concatenate)(w397, w399) -> (w395:sgl[])
            n198 = Build Array (concatenate)(w396, w398) -> (w394:sgl[])
            n199 = global write "VAR总磷总氮全局变量.vi" "波形图-消解温度"(w395) -> ()
            n200 = global write "VAR总磷总氮全局变量.vi" "波形图-注射器温度"(w394) -> ()
          }
          frame True {
            w400 = dbl[] [] ("波形图-消解温度")
            n201 = global write "VAR总磷总氮全局变量.vi" "波形图-消解温度"(w400) -> ()
            n202 = global write "VAR总磷总氮全局变量.vi" "波形图-注射器温度"(w400) -> ()
          }
        }
      }
    }
  }
  n203 = while {
    shift-right: [w401] -> _
    shift-left: _ -> [w406]
    tunnel: w8 -> [w404]
    stop <- FALSE stop-if-true
    n204 = File/Directory Info(path=w404) -> (last mod=w401:timestamp, error out=w402:errorcluster)  [unwired: 1 in, 5 out]
    n205 = Wait (ms)(milliseconds to wait=u32 1000 ("等待时间（毫秒）")) -> ()  [unwired: 1 out]
    n206 = Not Equal?(x=w406, y=w401) -> (x != y?=w405:bool)
    n207 = case shown="True" w405 {
      tunnel: [_ w408] -> _
      tunnel: w402 -> [_ _]
      frame False {
      }
      frame True {
        n208 = call "配置初始化.vi"() -> ("error out"=w408:errorcluster)  [unwired: 11 in]
      }
    }
  }
  n209 = flat-sequence {
    tunnel: w7 -> [_]
    frame #0 {
      (unwired) u32 0 ("等待时间（毫秒）")
      n210 = control-ref of="周期设置"() -> (w413:refnum<vi>)
      n211 = call "试剂余量后台任务.vi"() -> ()  [unwired: 12 in]
      n212 = call "New TimingControl.vi"("Reference"=w413) -> ("error out"=w411:errorcluster, "TimingControl out"=w412:refnum<class "TimingControl.lvclass">)  [unwired: 9 in]
      n213 = call "taskqueue ref.vi"() -> ("队列输出"=w414:refnum<queue>)  [unwired: 10 in, 1 out]
      n214 = while {
        tunnel: w414 -> [w433]
        shift-right: [w426] -> w410
        shift-left: w412 -> [w431]
        shift-right: [w425] -> w409
        shift-left: w411 -> [w430]
        stop <- FALSE stop-if-true
        n215 = global read "VAR总磷总氮全局变量.vi" "状态告警区"() -> (w434:T4)
        n216 = Wait (ms)(milliseconds to wait=u32 500 ("等待时间（毫秒）")) -> ()  [unwired: 1 out]
        n217 = global read "model config var.vi" "启动队列名称"() -> (w420:cluster{"String":string, "Value":u16}[])
        n218 = Unbundle By Name(w434) -> ("工作状态"=w432:u16, "系统时间"=w428:timestamp)
        n219 = for {
          tunnel: w420 -> [w445] mode=indexing
          tunnel: [w444] -> w419 mode=indexing
          n220 = Unbundle By Name(w445) -> ("String"=w444:string)
        }
        n221 = case shown="1, Default" w432 {
          tunnel: [FALSE TRUE] -> w427
          frame 0 {
          }
          frame 1, Default {
          }
        }
        n222 = property class="TimingControl"(reference=w431, error in=w430, "Properties:仪器时间"=w428, "Properties:仪器运行状态"=w427) -> (reference out=w426:refnum<class "TimingControl.lvclass">, error out=w425:errorcluster, "Properties:命令输出"=w429:cluster{"启动":bool, "控制命令":T12, "测量参数":T13})
        n223 = Array To Spreadsheet String(delimiter (Tab)="/" ("分隔符(Tab)"), array=w419, 3:"" ("格式字符串")) -> (spreadsheet string=w422:string)
        n224 = Unbundle By Name(w429) -> ("启动"=w416:bool, "控制命令"=w418:T12)
        n225 = Insert Into Array(array=w419, new element=w422) -> (w421:string[])  [unwired: 1 in]
        n226 = Bundle(w421) -> ()  [unwired: 1 in, 1 out]
        n227 = Bundle("控制命令"=w418, "") -> (w417:cluster{"控制命令":T12, string})  [unwired: 1 in]
        n228 = case shown="True" w416 {
          tunnel: w417 -> [_ w438]
          tunnel: w433 -> [_ w441]
          frame False {
          }
          frame True {
            n229 = Get Queue Status(queue=w441) -> (queue out=w439:refnum<queue>, # elements in queue=w440:i32)  [unwired: 2 in, 6 out]
            n230 = Equal To 0?(x=w440) -> (x = 0?=w437:bool)
            n231 = case shown="True" w437 {
              tunnel: w439 -> [_ w443]
              tunnel: w438 -> [_ w442]
              frame False {
              }
              frame True {
                n232 = Enqueue Element(queue=w443, element=w442) -> ()  [unwired: 2 in, 3 out]
              }
            }
          }
        }
      }
      n233 = call "task.vi"() -> ()  [unwired: 12 in]
      n234 = call "Close TimingControl.vi"("error in (no error)"=w409, "TimingControl in"=w410) -> ()  [unwired: 9 in, 1 out]
    }
  }
  n235 = while {
    tunnel: w7 -> [_]
    stop <- FALSE stop-if-true
    n236 = flat-sequence {
      frame #0 {
        n237 = global read "model config var.vi" "启动队列名称"() -> (w449:cluster{"String":string, "Value":u16}[])
        n238 = for {
          tunnel: w449 -> [w457] mode=indexing
          shift-right: [w456] -> w452
          shift-left: "" -> [w455]
          tunnel: [w454] -> w450 mode=indexing
          n239 = Unbundle By Name(w457) -> ("String"=w454:string)
          n240 = Concatenate Strings(w455, w454) -> (w456:string)
        }
        n241 = property on="单选按钮" class="RadioBtnsControl (strict)"() -> ("Controls[]"=w451:refnum<vi>[])  [unwired: 2 in, 2 out]
        n242 = global write "VAR总磷总氮全局变量.vi" "模块名称"(w452) -> ()
        n243 = for {
          tunnel: w451 -> [w465] mode=indexing
          tunnel: w450 -> [w464]
          n244 = property class="Ctl"(reference=w465) -> (reference out=w463:refnum<vi>, "Label.Text"=w459:string)  [unwired: 1 in, 1 out]
          n245 = case shown="\"COD\"" w459 {
            selector: w459 -> [w466 _]
            tunnel: [w466 "CODcr"] -> w458
            frame Default {
            }
            frame "COD" {
            }
          }
          n246 = Search 1D Array(1D array=w464, element=w458) -> (index of element=w462:i32)  [unwired: 1 in]
          n247 = Not Equal?(x=w462, y=-1) -> (x != y?=w460:bool)
          n248 = property class="Ctl"(reference=w463, "Visible"=w460) -> ()  [unwired: 1 in, 2 out]
        }
      }
      frame #1 {
        n249 = Wait (ms)(milliseconds to wait=u32 1000 ("等待时间（毫秒）")) -> ()  [unwired: 1 out]
      }
    }
  }
  n250 = call "时间延迟"("error in (no error)"=w6) -> ("error out"=w26:errorcluster)  [unwired: 10 in]
  n251 = vi-ref "斯坦道总磷总氮.lvlib:校准设置页.vi"() -> (w15:refnum<vi>)
  n252 = vi-ref "斯坦道总磷总氮.lvlib:参数设置页.vi"() -> (w19:refnum<vi>)
  n253 = property class="VI"(reference=w15, error in=w10) -> (reference out=w13:refnum<vi>, "Exec.State"=w14:T14)  [unwired: 1 out]
  n254 = property class="VI"(reference=w19, error in=w11) -> (reference out=w17:refnum<vi>, "Exec.State"=w18:T14)  [unwired: 1 out]
  n255 = while {
    tunnel: w26 -> [_]
    stop <- FALSE stop-if-true
    n256 = Wait (ms)(milliseconds to wait=u32 1000 ("等待时间（毫秒）")) -> ()  [unwired: 1 out]
    n257 = global read "VAR总磷总氮全局变量.vi" "状态告警区"() -> (w494:T4)
    n258 = global read "VAR总磷总氮全局变量.vi" "状态告警区"() -> (w495:T4)
    n259 = global read "VAR总磷总氮全局变量.vi" "状态告警区"() -> (w493:T4)
    n260 = global read "VAR总磷总氮全局变量.vi" "状态告警区"() -> (w491:T4)
    n261 = Unbundle By Name(w495) -> ("F0"=→"F0":sgl, "F1"=→"F1":sgl, "F2"=→"F2":sgl, "F3"=→"F3":sgl, "ADC"=→"ADC":sgl, "总磷控温温度1"=→"消解温度":sgl, "营养盐控温温度2"=→"注射器温度":sgl)
    n262 = Unbundle By Name(w494) -> ("日志代码"=w469:u16)
    "步骤" <- w469
    n263 = Unbundle By Name(w491) -> ("日志代码"=w490:u16)
    n264 = Unbundle By Name(w493) -> ("flowid"=w473:u16, "工作状态"=w486:u16, "id"=w487:u16)
    n265 = case shown="0" w486 {
      frame 0 {
        n266 = local write "数组"(string[] [] ("数组")) -> ()
      }
      frame 1, Default {
      }
    }
    n267 = feedback #4() -> (w492:u16)  [unwired: 1 in]
    n268 = feedback-in #4(w490) -> ()
    n269 = Not Equal To 0?(x=w486) -> (x != 0?=w471:bool)
    n270 = property on="总步数" class="DigNum (strict)"() -> ("Value"=w476:i32)  [unwired: 2 in, 2 out]
    n271 = Divide(x=w469, y=w476) -> (x/y=w475:dbl)
    n272 = Not Equal?(x=w490, y=w492) -> (x != y?=w489:bool)
    n273 = call <vilib>:"Boolean Crossing PtByPt.vi"("direction"=enum16{"either", "false-true", "true-false"}."either", "input"=w471) -> ("crossing"=w484:bool)  [unwired: 1 in]
    n274 = feedback-in #5(w469) -> ()
    n275 = feedback #5() -> (w497:u16)  [unwired: 1 in]
    n276 = Subtract(x=w469, y=1) -> (x-y=→"多列列表框":i32)
    n277 = case shown="True" w484 {
      tunnel: w487 -> [_ w520]
      tunnel: w473 -> [_ w508]
      tunnel: w471 -> [_ w506]
      frame False {
      }
      frame True {
        n278 = global read "VAR总磷总氮全局变量.vi" "最近一次工作状态"() -> (w507:u16)
        n279 = case shown="3" w507 {
          selector: w507 -> [w526 _ _ _ _ _ _ _ _ _ _ _]
          tunnel: [w525 "【水样测试】" ("字符串") w529 "【零点核查】" ("字符串") "【跨度核查】" ("字符串") "【空白测试】" ("字符串") "【平行样测试】" ("字符串") "【加标回收】" ("字符串") "【空白校准】" ("字符串") "【标样校准】" ("字符串") "【单步调试】" ("字符串") "【简易流程】" ("字符串")] -> w501
          tunnel: w508 -> [_ _ w528 _ _ _ _ _ _ _ _ _]
          frame 0, Default {
            n280 = Number To Decimal String(number=w526) -> (decimal integer string=w525:string)  [unwired: 1 in]
          }
          frame 1 {
          }
          frame 2 {
            n281 = case shown="0, Default" w528 {
              tunnel: ["【标样核查】" ("字符串") "【快捷测试】" ("字符串")] -> w529
              frame 0, Default {
              }
              frame 5 {
              }
            }
          }
          frame 3 {
          }
          frame 4 {
          }
          frame 5 {
          }
          frame 6 {
          }
          frame 7 {
          }
          frame 8 {
          }
          frame 9 {
          }
          frame 254 {
          }
          frame 255 {
          }
        }
        n282 = global read "VAR总磷总氮全局变量.vi" "状态告警区"() -> (w518:T4)
        n283 = Concatenate Strings("<<" ("字符串"), w501, "启动" ("字符串")) -> (w500:string)
        n284 = Unbundle By Name(w518) -> ("F0"=w517:sgl, "F1"=w516:sgl, "F2"=w515:sgl, "F3"=w514:sgl, "id"=w513:u16, "flowid"=w512:u16, "量程"=w511:u16)
        n285 = Concatenate Strings(w501, "停止>>" ("字符串")) -> (w504:string)
        n286 = Format Into String(format string="F0=%#f,F1=%#f,F2=%#f,F3=%#f,Flow=%d-%-d-%-d" ("格式字符串"), w517, w516, w515, w514, w513, w512, w511) -> (resulting string=w509:string)  [unwired: 2 in, 1 out]
        n287 = Select(t=w500, s=w506, f=w504) -> (s? t:f=w505:string)
        n288 = call "id参数转换.vi"("id"=w520) -> ("table输出"=w519:string)  [unwired: 9 in, 1 out]
        n289 = Get Date/Time In Seconds() -> (seconds since 1Jan1904=w523:timestamp)
        n290 = Bundle By Name(cluster=T15 {"时间标识"=timestamp(0 s since 1904-01-01), "设备"="", "日志信息"="", "流程参数"=""} ("data in"), "时间标识"=w523, "设备"=w519, "日志信息"=w505, "流程参数"=w509) -> (w522:T15)
        n291 = call "总磷总氮操作日志.vi"("data in"=w522) -> ()  [unwired: 10 in, 1 out]
      }
    }
    n292 = case shown="True" w489 {
      frame False {
      }
      frame True {
        n293 = property on="多列列表框" class="MCListbox (strict)"() -> ("ItemNames"=w546:string[][], "Value"=w542:i32)  [unwired: 2 in, 2 out]
        n294 = Index Array(array=w546, index (row)=w542) -> (element=w545:string[])  [unwired: 1 in]
        n295 = Index Array(array=w545) -> (element=w544:string)  [unwired: 1 in]
        n296 = call "过滤筛选流程.vi"("字符串"=w544) -> ("匹配后偏移量"=w543:i32)  [unwired: 10 in]
        n297 = case shown="Default" w543 {
          tunnel: w544 -> [w548 _]
          tunnel: w542 -> [w547 _]
          frame Default {
            n298 = case shown="\"读数\"" w548 {
              selector: w548 -> [w554 w561]
              tunnel: [w554 w561] -> w550
              tunnel: [string[] [] ("数组") w556] -> w549
              tunnel: w547 -> [_ w560]
              frame "读数" {
              }
              frame Default {
                n299 = Equal?(x=w560, y=1) -> (x = y?=w558:bool)
                n300 = Select(t=string[] [], s=w558, f="数组") -> (s? t:f=w556:string[])
              }
            }
            n301 = for {
              N: 1 -> [_]
              tunnel: w550 -> [w563]
              shift-right: [w562] -> w551
              shift-left: w549 -> [w564]
              n302 = Search 1D Array(1D array=w564, element=w563) -> (index of element=w567:i32)  [unwired: 1 in]
              n303 = Format Into String(format string="%s" ("格式字符串"), w563) -> (resulting string=w568:string)  [unwired: 2 in, 1 out]
              n304 = Equal?(x=w567, y=-1) -> (x = y?=w565:bool)
              n305 = case shown="True" w565 {
                tunnel: w568 -> [_ w578]
                tunnel: w564 -> [w570 w582]
                tunnel: w563 -> [_ w581]
                tunnel: [w570 w580] -> w562
                frame False {
                }
                frame True {
                  n306 = Insert Into Array(array=w582, new element=w581) -> (w580:string[])  [unwired: 1 in]
                  n307 = global read "VAR总磷总氮全局变量.vi" "状态告警区"() -> (w577:T4)
                  n308 = Unbundle By Name(w577) -> ("工作状态"=w576:u16, "flowid"=w571:u16)
                  n309 = case shown="2" w576 {
                    selector: w576 -> [w597 _ _ _ _ _ _ _ _ _ _ _]
                    tunnel: [w596 "【水样测试】" ("字符串") w600 "【零点核查】" ("字符串") "【跨度核查】" ("字符串") "【空白测试】" ("字符串") "【平行样测试】" ("字符串") "【加标回收】" ("字符串") "【空白校准】" ("字符串") "【标样校准】" ("字符串") "【单步调试】" ("字符串") w611] -> w574
                    tunnel: w571 -> [_ _ w599 _ _ _ _ _ _ _ _ _]
                    frame 0, Default {
                      n310 = Number To Decimal String(number=w597) -> (decimal integer string=w596:string)  [unwired: 1 in]
                    }
                    frame 1 {
                    }
                    frame 2 {
                      n311 = case shown="5" w599 {
                        tunnel: ["【标样核查】" ("字符串") "【快捷测试】" ("字符串")] -> w600
                        frame Default {
                        }
                        frame 5 {
                        }
                      }
                    }
                    frame 3 {
                    }
                    frame 4 {
                    }
                    frame 5 {
                    }
                    frame 6 {
                    }
                    frame 7 {
                    }
                    frame 8 {
                    }
                    frame 9 {
                    }
                    frame 254 {
                    }
                    frame 255 {
                      n312 = local read "简易步骤名称"() -> (w613:string)
                      n313 = Format Into String(format string="(%s)" ("格式字符串"), initial string="【简易流程】" ("工作状态"), w613) -> (resulting string=w611:string)  [unwired: 1 in, 1 out]
                    }
                  }
                  n314 = global read "VAR总磷总氮全局变量.vi" "状态告警区"() -> (w595:T4)
                  n315 = global read "VAR总磷总氮全局变量.vi" "状态告警区"() -> (w592:T4)
                  n316 = Unbundle By Name(w592) -> ("F0"=w589:sgl, "F1"=w588:sgl, "F2"=w587:sgl, "F3"=w586:sgl, "id"=w585:u16, "flowid"=w584:u16, "量程"=w583:u16)
                  n317 = Unbundle By Name(w595) -> ("id"=w573:u16)
                  n318 = call "id参数转换.vi"("id"=w573) -> ("table输出"=w572:string)  [unwired: 9 in, 1 out]
                  n319 = Concatenate Strings(w574, w578) -> (w575:string)
                  n320 = Format Into String(format string="F0=%#f,F1=%#f,F2=%#f,F3=%#f,Flow=%d-%-d-%-d" ("格式字符串"), w589, w588, w587, w586, w585, w584, w583) -> (resulting string=w590:string)  [unwired: 2 in, 1 out]
                  n321 = Get Date/Time In Seconds() -> (seconds since 1Jan1904=w593:timestamp)
                  n322 = Bundle By Name(cluster=T15 {"时间标识"=timestamp(0 s since 1904-01-01), "设备"="", "日志信息"="", "流程参数"=""} ("data in"), "时间标识"=w593, "设备"=w572, "日志信息"=w575, "流程参数"=w590) -> (w594:T15)
                  n323 = call "总磷总氮操作日志.vi"("data in"=w594) -> ()  [unwired: 10 in, 1 out]
                }
              }
            }
            n324 = local write "数组"(w551) -> ()
          }
          frame -1 {
          }
        }
      }
    }
    n325 = Not Equal?(x=w469, y=w497) -> (x != y?=w496:bool)
    n326 = Multiply(x=w475, y=100.0) -> (x*y=w472:dbl)
    "滑动杆" <- w472
    n327 = case shown="True" w496 {
      tunnel: w469 -> [_ w617]
      frame False {
      }
      frame True {
        n328 = Subtract(x=w617, y=1) -> (x-y=w615:i32)
        n329 = Subtract(x=w615, y=5) -> (x-y=w619:i32)
        n330 = Greater Or Equal To 0?(x=w619) -> (x >= 0?=w618:bool)
        n331 = property on="多列列表框" class="MCListbox (strict)"() -> (error out=w623:errorcluster, "TopLeft"=w624:T16)  [unwired: 2 in, 1 out]
        n332 = Select(t=w619, s=w618, f=0) -> (s? t:f=w620:i32)
        n333 = Bundle By Name(cluster=w624, "Row"=w620) -> (w625:T16)
        n334 = property on="多列列表框" class="MCListbox (strict)"(error in=w623, "TopLeft"=w625) -> ()  [unwired: 1 in, 2 out]
      }
    }
    n335 = global write "VAR总磷总氮全局变量.vi" "测试进度"(w472) -> ()
  }
  n336 = case shown="\"Idle\"" w14 {
    tunnel: w13 -> [w626 w630]
    tunnel: [w626 w627] -> w12
    frame "Bad", Default {
    }
    frame "Idle" {
      n337 = invoke class="VI" method="Run VI"(reference=w630, "Wait until done"=FALSE ("结束前等待"), "Auto Dispose Ref"=TRUE ("自动销毁引用")) -> (reference out=w627:refnum<vi>)  [unwired: 2 in, 4 out]
    }
  }
  n338 = case shown="\"Idle\"" w18 {
    tunnel: w17 -> [w631 w635]
    tunnel: [w631 w632] -> w16
    frame "Bad", Default {
    }
    frame "Idle" {
      n339 = invoke class="VI" method="Run VI"(reference=w635, "Wait until done"=FALSE ("结束前等待"), "Auto Dispose Ref"=TRUE ("自动销毁引用")) -> (reference out=w632:refnum<vi>)  [unwired: 2 in, 4 out]
    }
  }
  n340 = Obtain Notifier(name (unnamed)=w20, notification data type=FALSE) -> (notifier out=w21:refnum<notifier>)  [unwired: 2 in, 2 out]
  n341 = Obtain Queue(name (unnamed)=w20, element data type=cluster{"命令":string, "data":variant} {"命令"="", "data"=variant}) -> (queue out=w23:refnum<queue>)  [unwired: 3 in, 2 out]
  n342 = while {
    tunnel: w23 -> [w639]
    tunnel: w21 -> [w638]
    tunnel: w16 -> [w637]
    tunnel: w12 -> [w636]
    stop <- FALSE stop-if-true
    n343 = event shown="[8] \"手动启动\": Value Change" {
      selector: _ -> [_ _ _ _ _ _ _ _ _ _ _ _ _ _]
      dyn-events: _ -> [_ _ _ _ _ _ _ _ _ _ _ _ _ _]
      timeout: _ -> [_ _ _ _ _ _ _ _ _ _ _ _ _ _]
      tunnel: w639 -> [_ _ _ _ _ _ _ _ w653 _ w660 _ _ _]
      tunnel: w638 -> [_ _ _ _ _ _ _ _ _ _ w659 _ _ _]
      tunnel: w637 -> [_ _ _ _ _ _ _ _ _ _ _ w680 _ _]
      tunnel: w636 -> [_ _ _ _ _ _ _ _ _ _ _ _ w686 _]
      event Timeout {
        n344 = event-data() -> ()  [unwired: 1 in, 3 out]
      }
      event "流程操作": Value Change {
        n345 = event-data() -> ()  [unwired: 1 in, 6 out]
        n346 = global read "总磷总氮断电保存全局变量.vi" "简易流程路径"() -> (w641:path)
        n347 = global read "总磷总氮断电保存全局变量.vi" "流程路径"() -> (w642:path)
        n348 = call "流程批量写入.vi"("简易流程路径"=w641, "添加的路径"=w642) -> ()  [unwired: 10 in]
      }
      event "温度曲线": Value Change {
        n349 = event-data() -> ()  [unwired: 1 in, 6 out]
        n350 = call "温度曲线显示.vi"() -> ()  [unwired: 12 in]
      }
      event "试剂余量": Value Change {
        n351 = event-data() -> ()  [unwired: 1 in, 6 out]
        n352 = call "试剂余量显示UI.vi"() -> ()  [unwired: 12 in]
      }
      event "灯值调整": Value Change {
        n353 = event-data() -> ()  [unwired: 1 in, 6 out]
        n354 = call "灯值调整对话框.vi"() -> ()  [unwired: 12 in]
      }
      event "布尔": Value Change {
        n355 = event-data() -> ("NewVal"=w643:bool)  [unwired: 1 in, 5 out]
        n356 = case shown="False" w643 {
          frame False {
            n357 = global write "VAR总磷总氮全局变量.vi" "权限等级"(enum16{"一级权限", "二级权限", "三级权限", "超级权限"}."一级权限" ("权限等级")) -> ()
          }
          frame True {
            n358 = global read "VAR总磷总氮全局变量.vi" "权限密码"() -> (w647:u32[])
            n359 = global read "VAR总磷总氮全局变量.vi" "权限等级"() -> (w645:enum16{"一级权限", "二级权限", "三级权限", "超级权限"})
            n360 = call "密码权限设置.vi"("权限输入"=w645, "权限密码"=w647) -> ("权限输出"=w646:enum16{"一级权限", "二级权限", "三级权限", "超级权限"})  [unwired: 9 in]
            n361 = global write "VAR总磷总氮全局变量.vi" "权限等级"(w646) -> ()
          }
        }
      }
      event "权限等级": Mouse Down {
        n362 = event-data() -> ()  [unwired: 1 in, 8 out]
        n363 = global read "VAR总磷总氮全局变量.vi" "权限密码"() -> (w650:u32[])
        n364 = global read "VAR总磷总氮全局变量.vi" "权限等级"() -> (w648:enum16{"一级权限", "二级权限", "三级权限", "超级权限"})
        n365 = call "密码权限设置.vi"("权限输入"=w648, "权限密码"=w650) -> ("权限输出"=w649:enum16{"一级权限", "二级权限", "三级权限", "超级权限"})  [unwired: 9 in]
        n366 = global write "VAR总磷总氮全局变量.vi" "权限等级"(w649) -> ()
      }
      event "外设固件": Value Change {
        n367 = event-data() -> ()  [unwired: 1 in, 6 out]
        n368 = call "流程固件设置对话框.vi"() -> ()  [unwired: 12 in]
      }
      event "手动启动": Value Change {
        n369 = event-data() -> ()  [unwired: 1 in, 6 out]
        n370 = call "总磷总氮启动参数对话框.vi"() -> ("确认"=w651:bool, "元素"=w652:cluster{"命令":string, "data":variant})  [unwired: 10 in]
        n371 = case shown="True" w651 {
          tunnel: w653 -> [_ w656]
          tunnel: w652 -> [_ w655]
          frame False {
          }
          frame True {
            n372 = Flush Queue(queue=w656) -> (queue out=w654:refnum<queue>)  [unwired: 1 in, 2 out]
            n373 = Enqueue Element(queue=w654, element=w655) -> ()  [unwired: 2 in, 3 out]
          }
        }
      }
      event "调试": Value Change {
        n374 = event-data() -> ()  [unwired: 1 in, 6 out]
        n375 = call "简易流程调试界面.vi"() -> ()  [unwired: 12 in]
      }
      event "停止": Value Change {
        n376 = event-data() -> ()  [unwired: 1 in, 6 out]
        n377 = Two Button Dialog(message="确认停止？" ("消息")) -> (T button?=w657:bool)  [unwired: 2 in]
        n378 = case shown="True" w657 {
          tunnel: w660 -> [_ w676]
          tunnel: w659 -> [_ w675]
          frame False {
          }
          frame True {
            n379 = Send Notification(notification=TRUE ("通知"), notifier=w675) -> ()  [unwired: 1 in, 2 out]
            n380 = global read "VAR总磷总氮全局变量.vi" "状态告警区"() -> (w670:T4)
            n381 = global read "VAR总磷总氮全局变量.vi" "状态告警区"() -> (w662:T4)
            n382 = Unbundle By Name(w670) -> ("id"=w669:u16)
            n383 = Unbundle By Name(w662) -> ("id"=w661:u16)
            n384 = Bundle By Name(cluster=T18 {"站号"=1, "量程切换"=enum."AUTO", "控制命令"=enum."停止测试", "模式设置"=enum."待机", "测量间隔"=0} ("参数"), "站号"=w669) -> (w671:T18)
            n385 = call "id参数转换.vi"("id"=w661) -> ("table输出"=w663:string)  [unwired: 9 in, 1 out]
            n386 = call "总磷总氮启动命令.vi"("参数"=w671) -> ("启动命令"=w672:cluster{"命令":string, "data":variant})  [unwired: 10 in]
            n387 = Get Date/Time In Seconds() -> (seconds since 1Jan1904=w666:timestamp)
            n388 = Bundle By Name(cluster=T17 {"时间"=timestamp(0 s since 1904-01-01), "参数"="", "日志信息"="", "流程参数"=""} ("data in"), "时间"=w666, "参数"=w663, "日志信息"="手动停止") -> (w667:T17)
            n389 = Enqueue Element(queue=w676, element=w672) -> (error out=w664:errorcluster)  [unwired: 2 in, 2 out]
            n390 = call "总磷总氮操作日志.vi"("错误输入（无错误）"=w664, "data in"=w667) -> ()  [unwired: 9 in, 1 out]
          }
        }
      }
      event "参数设置", "参数查询": Value Change {
        n391 = event-data() -> ()  [unwired: 1 in, 6 out]
        n392 = invoke on="子面板" class="SubPnl" method="Remove VI"() -> (error out=w681:errorcluster)  [unwired: 3 in, 2 out]
        n393 = property on="仪器校准" class="Bool"("Visible"=TRUE ("可见")) -> ()  [unwired: 2 in, 2 out]
        n394 = property on="参数查询" class="Bool"("Visible"=FALSE ("可见")) -> ()  [unwired: 2 in, 2 out]
        n395 = property on="窗格" class="Pane"("Origin"=T3 {"Horizontal"=0, "Vertical"=640} ("原点")) -> ()  [unwired: 2 in, 2 out]
        n396 = invoke on="子面板" class="SubPnl" method="Insert VI"(error in=w681, "VI Ref"=w680) -> ()  [unwired: 2 in, 4 out]
        n397 = global write "VAR总磷总氮全局变量.vi" "页面"(enum16{"主页", "参数页", "校准页"}."参数页" ("页面")) -> ()
      }
      event "仪器校准": Value Change {
        n398 = event-data() -> ()  [unwired: 1 in, 6 out]
        n399 = invoke on="子面板" class="SubPnl" method="Remove VI"() -> (error out=w687:errorcluster)  [unwired: 3 in, 2 out]
        n400 = property on="仪器校准" class="Bool"("Visible"=FALSE ("可见")) -> ()  [unwired: 2 in, 2 out]
        n401 = property on="参数查询" class="Bool"("Visible"=TRUE ("可见")) -> ()  [unwired: 2 in, 2 out]
        n402 = global write "VAR总磷总氮全局变量.vi" "页面"(enum16{"主页", "参数页", "校准页"}."校准页" ("页面")) -> ()
        n403 = invoke on="子面板" class="SubPnl" method="Insert VI"(error in=w687, "VI Ref"=w686) -> ()  [unwired: 2 in, 4 out]
      }
      event "返回": Value Change {
        n404 = event-data() -> ()  [unwired: 1 in, 6 out]
        n405 = global write "VAR总磷总氮全局变量.vi" "页面"(enum16{"主页", "参数页", "校准页"}."主页" ("页面")) -> ()
        n406 = property on="窗格" class="Pane"("Origin"=T3 {"Horizontal"=0, "Vertical"=0} ("原点")) -> ()  [unwired: 2 in, 2 out]
      }
    }
  }
  n407 = while {
    tunnel: w23 -> [w701]
    stop <- FALSE stop-if-true
    n408 = Wait (ms)(milliseconds to wait=u32 1000 ("等待时间（毫秒）")) -> ()  [unwired: 1 out]
    n409 = global read "总磷总氮断电保存全局变量.vi" "MB通信方式选择"() -> (w699:enum16{"串口", "TCP"})
    n410 = global read "VAR总磷总氮全局变量.vi" "升级固件关闭心跳包"() -> (w693:bool)
    n411 = global read "VAR总磷总氮全局变量.vi" "MB session in"() -> (w697:refnum<class "MB_Master.lvclass">)
    n412 = case shown="\"串口\", Default" w699 {
      tunnel: [w704 w705] -> w698
      frame "串口", Default {
        n413 = global read "总磷总氮断电保存全局变量.vi" "VISA Resource"() -> (w704:refnum<visa-resource-name>)
      }
      frame "TCP" {
        n414 = global read "总磷总氮断电保存全局变量.vi" "IP"() -> (w705:string)
      }
    }
    "字符串 2" <- w698
    n415 = property class="MB_Master"(reference=w697) -> ("Properties:Session Valid"=w695:bool)  [unwired: 1 in, 2 out]
    n416 = Not(x=w693) -> (.not. x?=w692:bool)
    n417 = Get Queue Status(queue=w701) -> (queue out=w700:refnum<queue>, # elements in queue=w696:i32)  [unwired: 2 in, 6 out]
    n418 = Equal To 0?(x=w696) -> (x = 0?=w690:bool)
    n419 = Compound Arithmetic op=AND ("复合运算")(w695, w692) -> (w694:bool)
    n420 = global write "VAR总磷总氮全局变量.vi" "心跳包打开状态"(w694) -> ()
    n421 = And(x=w690, y=w694) -> (x .and. y?=w691:bool)
    n422 = case shown="True" w691 {
      tunnel: w700 -> [_ w724]
      frame False {
      }
      frame True {
        n423 = global read "VAR总磷总氮全局变量.vi" "MB session in"() -> (w712:refnum<class "MB_Master.lvclass">)
        n424 = property class="MB_Master"(reference=w712) -> ("Properties:Session Valid"=w710:bool)  [unwired: 1 in, 2 out]
        n425 = global read "VAR总磷总氮全局变量.vi" "通讯状态"() -> (w713:bool)
        n426 = case shown="True" w710 {
          tunnel: [_ w726] -> w709
          frame False {
          }
          frame True {
            n427 = global read "VAR总磷总氮全局变量.vi" "MB session in"() -> (w725:refnum<class "MB_Master.lvclass">)
            n428 = call "版本号读取.vi"("MB session in"=w725) -> ("error out"=w726:errorcluster, "固件版本号"=w727:string)  [unwired: 8 in, 1 out]
            "固件版本号" <- w727
            n429 = global write "VAR总磷总氮全局变量.vi" "固件版本号"(w727) -> ()
          }
        }
        n430 = And(x=w710, y=w713) -> (x .and. y?=w711:bool)
        n431 = case shown="True" w711 {
          tunnel: [_ w728] -> w708
          tunnel: w709 -> [_ w729]
          frame False {
          }
          frame True {
            n432 = global read "VAR总磷总氮全局变量.vi" "MB session in"() -> (w731:refnum<class "MB_Master.lvclass">)
            n433 = call "序列号读取.vi"("Error in"=w729, "MB session in"=w731) -> ("error out"=w728:errorcluster, "序列号"=w730:string)  [unwired: 7 in, 1 out]
            n434 = global write "VAR总磷总氮全局变量.vi" "序列号"(w730) -> ()
          }
        }
        n435 = global read "model config var.vi" "启动队列名称"() -> (w715:cluster{"String":string, "Value":u16}[])
        n436 = for {
          tunnel: [w742] -> w716 mode=indexing
          tunnel: w715 -> [w743] mode=indexing
          tunnel: w708 -> [_]
          n437 = Unbundle By Name(w743) -> ("Value"=w742:u16)
        }
        n438 = for {
          shift-right: [w732] -> w718
          shift-left: w724 -> [w738]
          tunnel: w716 -> [w733] mode=indexing
          n439 = Bundle By Name(cluster=cluster{"命令":string, "data":variant} {"命令"="", "data"=variant} ("元素"), "命令"="读状态告警区", "data"=w733) -> (w740:cluster{"命令":string, "data":variant})
          n440 = Bundle By Name(cluster=cluster{"命令":string, "data":variant} {"命令"="", "data"=variant} ("元素"), "命令"="读测量数据区", "data"=w733) -> (w735:cluster{"命令":string, "data":variant})
          n441 = Enqueue Element(queue=w738, element=w740) -> (queue out=w734:refnum<queue>)  [unwired: 2 in, 2 out]
          n442 = Enqueue Element At Opposite End(queue=w734, element=w735) -> (queue out=w732:refnum<queue>)  [unwired: 2 in, 2 out]
        }
        n443 = global read "VAR总磷总氮全局变量.vi" "状态告警区"() -> (w717:T4)
        n444 = Unbundle By Name(w717) -> ("系统时间"=w706:timestamp)
        n445 = Get Date/Time In Seconds() -> (seconds since 1Jan1904=w723:timestamp)
        n446 = Subtract(x=w723, y=w706) -> (x-y=w722:dbl)
        n447 = Absolute Value(x=w722) -> (abs(x)=w721:dbl)
        n448 = global read "VAR总磷总氮全局变量.vi" "通讯状态"() -> (w707:bool)
        n449 = Greater Or Equal?(x=w721, y=30.0) -> (x >= y?=w719:bool)
        n450 = Compound Arithmetic op=AND ("复合运算")(w719, w707) -> (w714:bool)
        n451 = case shown="True" w714 {
          tunnel: w718 -> [_ w745]
          frame False {
          }
          frame True {
            n452 = call "总磷总氮启动命令.vi"("参数"=T18 {"站号"=3, "量程切换"=enum."AUTO", "控制命令"=enum."校时", "模式设置"=enum."待机", "测量间隔"=0}) -> ("启动命令"=w744:cluster{"命令":string, "data":variant})  [unwired: 10 in]
            n453 = Enqueue Element(queue=w745, element=w744) -> ()  [unwired: 2 in, 3 out]
          }
        }
      }
    }
  }
